vi "GetClassPath.vi"(8 "error in":errorcluster, 10 "class name":string, 11 "Repository in":refnum<class "modification container.lvclass">) -> (0 "error out":errorcluster, 2 "class path":path, 3 "Repository out":refnum<class "modification container.lvclass">)   [LabVIEW 2013, in "modification container.lvclass"]
doc: "Gets the path to the Class based on the Class Name. \nThe default behavior is build the path of the class on top of the class folder path. The name of the class and the folder it contains needs to be the same. A simple lookup from index and name would be the other option."
uses:
  modification container.lvclass
  collection/available modifications.vi
  collection/VI modification collection.lvclass
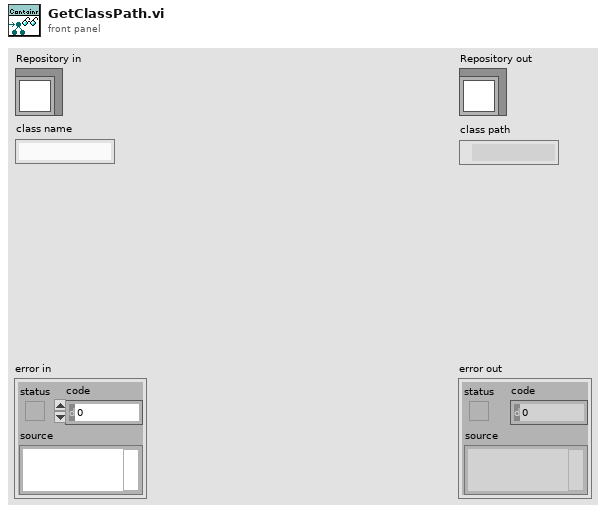
[diagram p1: front panel]
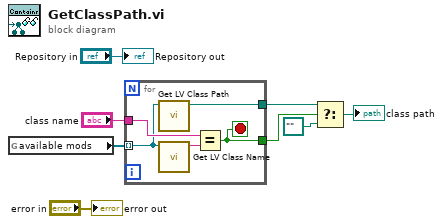
[diagram p0: block diagram]
diagram:
  n1 = global read "available modifications.vi" "available mods"() -> (w6:refnum<class "VI modification.lvclass">[])
  n2 = for {
    tunnel: w6 -> [w11] mode=indexing
    tunnel: "class name" -> [w12]
    tunnel: [w10] -> w3
    tunnel: [w9] -> w4
    stop <- w9 stop-if-true
    n3 = call <vilib>:"Get LV Class Path.vi"("object"=w11) -> ("class path"=w10:path)  [unwired: 9 in, 1 out]
    n4 = call <vilib>:"Get LV Class Name.vi"("object"=w11) -> ("class name"=w13:string)  [unwired: 9 in, 1 out]
    n5 = Equal?(x=w12, y=w13) -> (x = y?=w9:bool)
  }
  n6 = Select(t=w3, s=w4, f=path "") -> (s? t:f=→"class path":path)
  "error out" <- "error in"
  "Repository out" <- "Repository in"
